vi "temp_FlpLib Perturbance.vi"(0 "freq":sgl, 1 "dT":sgl, 5 "amplitude":sgl) -> (4 "Perturbance":sgl)   [LabVIEW 2016]
uses:
  Calculus/Integrator/FlpLib Integrator 0.vi
  <userlib>/_NI FLP Library/FPGA/outsideSCTL/FlpLib Subtract Shared Instance 0.vi
  <userlib>/_NI FLP Library/FPGA/outsideSCTL/FlpLib Greater Than Shared Instance 0.vi
  <userlib>/_NI FLP Library/FPGA/outsideSCTL/FlpLib Sine Shared Instance 0.vi
  <userlib>/_NI FLP Library/FPGA/outsideSCTL/FlpLib Multiply Shared Instance 0.vi
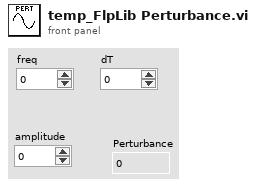
[diagram p1: front panel]
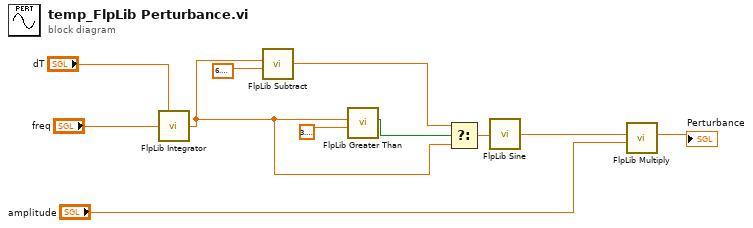
[diagram p0: block diagram]
diagram:
  n1 = call-poly "FlpLib Integrator.vi"("dt"="dT", "dx"="freq") -> ("x"=w1:sgl)  [unwired: 13 in]
  n2 = call-poly <userlib>:"FlpLib Subtract.vi"("y"=sgl 6.2831855, "x"=w1) -> ("x-y"=w3:sgl)  [unwired: 5 in]
  n3 = call-poly <userlib>:"FlpLib Greater Than.vi"("y"=sgl 3.1415927, "x"=w1) -> ("x > y?"=w7:bool)  [unwired: 5 in]
  n4 = Select(t=w3, s=w7, f=w1) -> (s? t:f=w8:sgl)
  n5 = call-poly <userlib>:"FlpLib Sine.vi"("x"=w8) -> ("sin(x)"=w9:sgl)  [unwired: 4 in]
  n6 = call-poly <userlib>:"FlpLib Multiply.vi"("y"="amplitude", "x"=w9) -> ("x*y"=→"Perturbance":sgl)  [unwired: 5 in]
